vi "UI_Queue_Dequeue.vi"(8 "error in (no error)":errorcluster, 9 "timeout in ms (-1)":i32=-1, 11 "UI Queue in":refnum<queue>) -> (0 "error out":errorcluster, 1 "Value":variant, 2 "Cmd":string, 3 "UI Queue out":refnum<queue>)   [LabVIEW 2016]
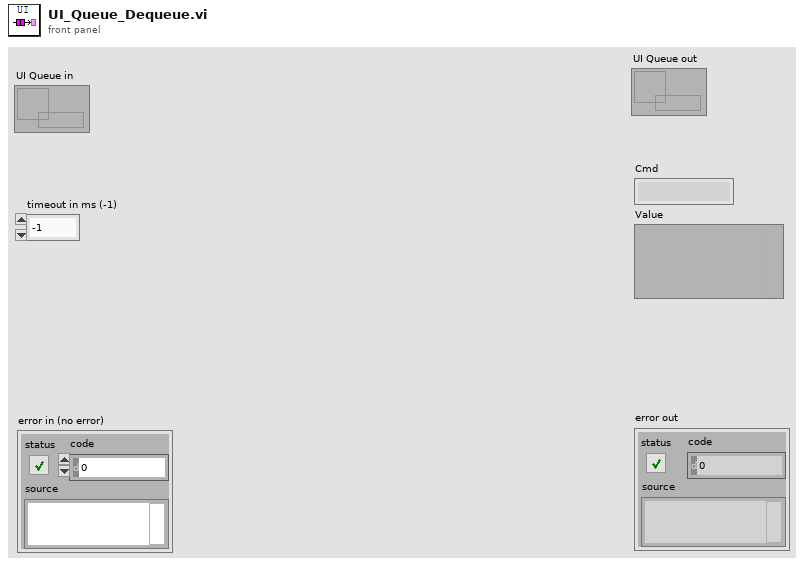
[diagram p1: front panel]
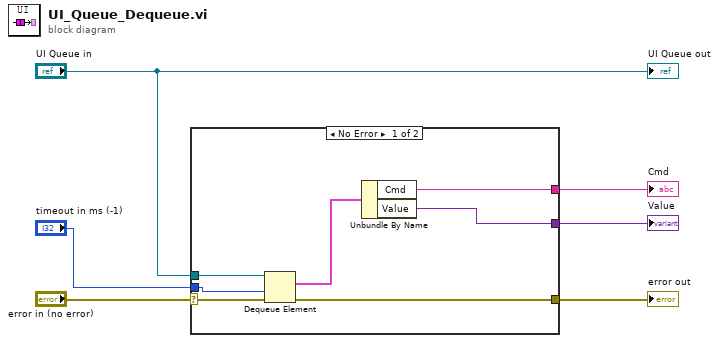
[diagram p0: block diagram]
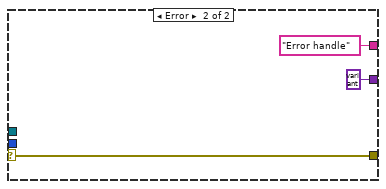
[diagram p2: hidden frame]
diagram:
  n1 = case shown="No Error" "error in (no error)" {
    selector: "error in (no error)" -> [w11 w16]
    tunnel: "UI Queue in" -> [w13 _]
    tunnel: [w10 w16] -> w4
    tunnel: [w9 "Error handle" ("Cmd")] -> w3
    tunnel: [w8 variant ("Value")] -> w2
    tunnel: "timeout in ms (-1)" -> [w7 _]
    frame No Error {
      n2 = Dequeue Element(queue=w13, timeout in ms (-1)=w7, error in (no error)=w11) -> (element=w12:cluster{"Cmd":string, "Value":variant}, error out=w10:errorcluster)  [unwired: 2 out]
      n3 = Unbundle By Name(w12) -> ("Cmd"=w9:string, "Value"=w8:variant)
    }
    frame Error {
    }
  }
  "error out" <- w4
  "Cmd" <- w3
  "Value" <- w2
  "UI Queue out" <- "UI Queue in"
